vi "4310 DMM Close and Stop Stream.vi"(7 "gRPCid":T1, 8 "error in (no error)":errorcluster, 10 "task in":refnum<k21>, 11 "IVI Refnum in":refnum<k15>) -> (0 "error out":errorcluster)   [LabVIEW 2019]
uses:
  VIs/grpcId.ctl
  VIs/gprc-support.lvlib
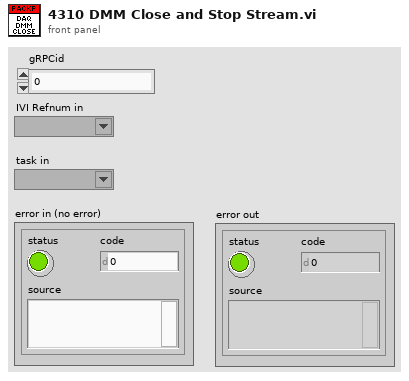
[diagram p1: front panel]
types:
  T1 = typedef "gprc-support.lvlib/grpcId.ctl" = u64
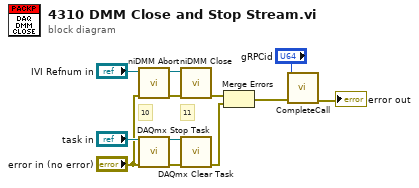
[diagram p0: block diagram]
diagram:
  # "10"
  # "11"
  n1 = call <instrlib>:"niDMM Abort.vi"("error in (no error)"="error in (no error)", "instrument handle"="IVI Refnum in") -> ("error out"=w6:errorcluster, "instrument handle out"=w5:refnum<k15>)  [unwired: 8 in]
  n2 = call <vilib>:"DAQmx Stop Task.vi"("task/channels in"="task in", "error in"="error in (no error)") -> ("task out"=w10:refnum<k21>, "error out"=w9:errorcluster)  [unwired: 12 in]
  n3 = call <instrlib>:"niDMM Close.vi"("error in (no error)"=w6, "instrument handle"=w5) -> ("error out"=w11:errorcluster)  [unwired: 9 in]
  n4 = call <vilib>:"DAQmx Clear Task.vi"("task in"=w10, "error in"=w9) -> ("error out"=w12:errorcluster)  [unwired: 13 in]
  n5 = Merge Errors(w11, w12) -> (w3:errorcluster)
  n6 = call "CompleteCall.vi"("gRPCid"="gRPCid", "error in (no error)"=w3) -> ("error out"=→"error out":errorcluster)  [unwired: 8 in]
